vi "EXCOM-25-EQ.vi"(0 "VISA resource name":refnum<visa-resource-name>, 2 "Bool Refnum":refnum<vi>, 3 "Display Equinox":dbl format="%.2f") -> (5 "OK Done":bool, 6 "HA":dbl format="%<%H:%M:%S%0u>t", 7 "Q String":string, 8 "RA":dbl format="%<%H:%M:%S%0u>t", 9 "Rotateur":dbl format="%.2f", 10 "DEC":dbl format="%<%H:%M:%S%0u>t", 11 "Dome":dbl format="%.2f", 12 "Epoque":dbl format="%.2f", 13 "Focus":dbl format="%.2f", 14 "VISA resource name dup":refnum<visa-resource-name>, 15 "Masse d'air":dbl format="%.2f", 16 "Temps Sidéral":dbl format="%<%H:%M:%S%0u>t", 17 "Temps Universel":dbl format="%<%H:%M:%S%0u>t", 18 "Année":dbl format="%.2f", 19 "Error OUT":errorcluster)   [LabVIEW 2011]
panel:
  out "Response":string
  in  "Error IN":errorcluster
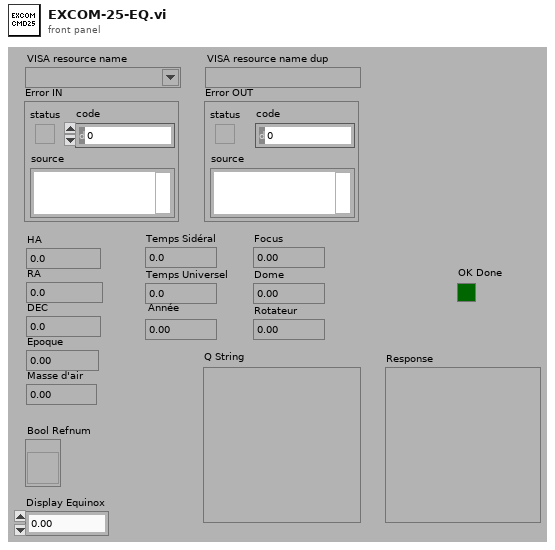
[diagram p1: front panel]
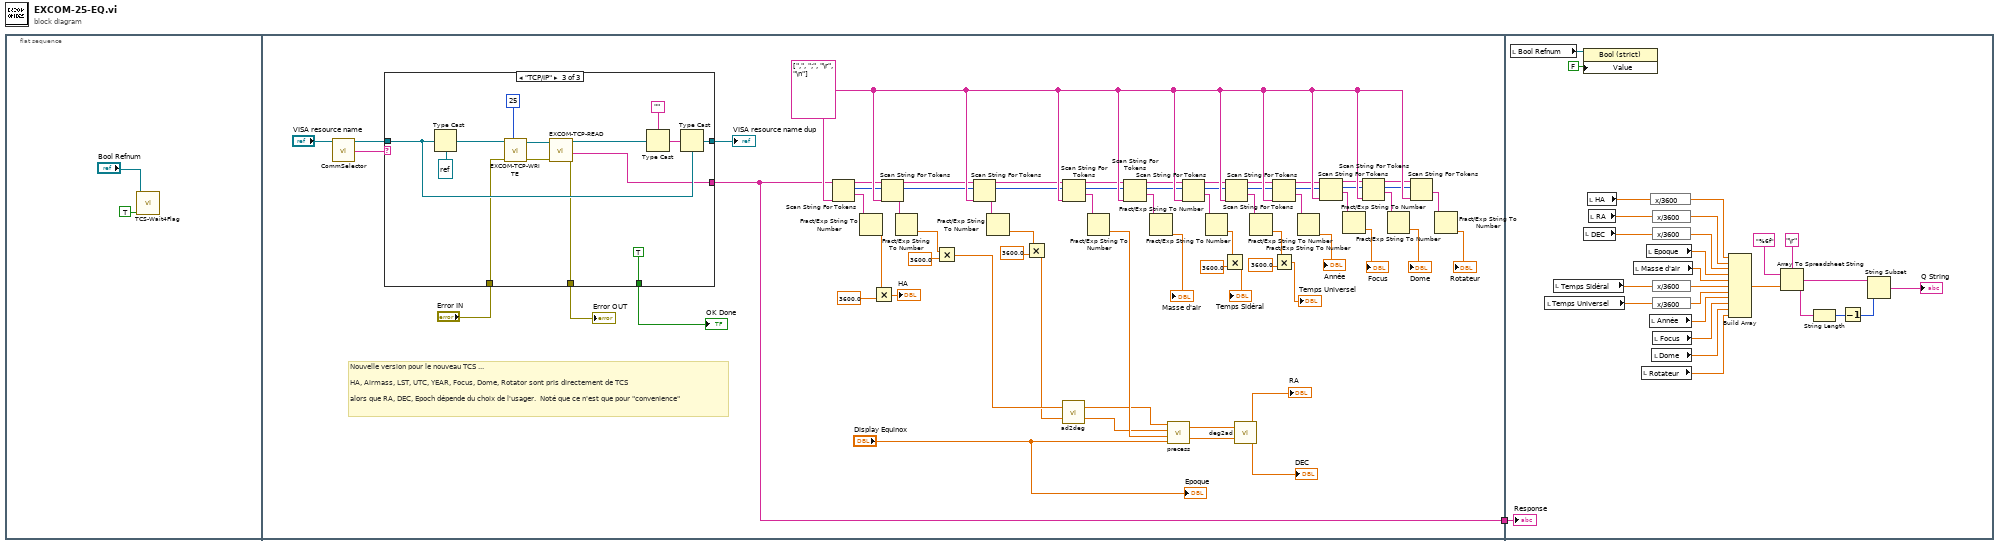
[diagram p0: block diagram]
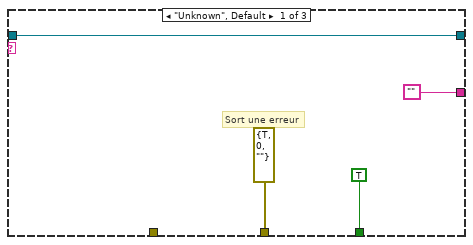
[diagram p2: hidden frame]
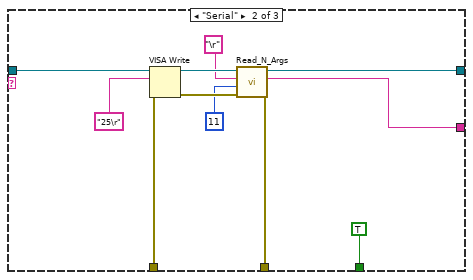
[diagram p3: hidden frame]
diagram:
  n1 = flat-sequence {
    tunnel: [w4] -> w1
    tunnel: w1 -> [w110]
    frame #0 {
      n2 = call "TCS-Wait4Flag.vi"("Raise Flag ?"=TRUE, "Ctl Refnum IN"="Bool Refnum") -> ()  [unwired: 8 in, 2 out]
    }
    frame #1 {
      w64 = string[] [",", ";", "\r", "\n"] ("delimiters (\\s,\\t,\\r,\\n)")
      # "Nouvelle version pour le nouveau TCS ...\n\nHA, Airmass, LST, UTC, YEAR, Focus, Dome, Rotator sont pris directement de TCS\n\nalors que RA, DEC, Epoch dépende du choix de l'usager.  Noté que ce n'est que pour \"convenience\""
      n3 = call "CommSelector.vi"("VISA resource name"="VISA resource name") -> ("VISA resource name"=w66:refnum<visa-resource-name>, "CommType"=w65:string)  [unwired: 13 in]
      n4 = case shown="\"TCP/IP\"" w65 {
        tunnel: w66 -> [w73 w78 w95]
        tunnel: [TRUE ("OK Done") TRUE ("OK Done") TRUE ("OK Done")] -> w71
        tunnel: [errorcluster {"status"=TRUE, "code"=0, "source"=""} ("error out") w85 w89] -> w70
        tunnel: [w73 w79 w94] -> w69
        tunnel: "Error IN" -> [_ w77 w90]
        tunnel: ["" w76 w87] -> w4
        frame "Unknown", Default {
          # "Sort une erreur"
        }
        frame "Serial" {
          n5 = VISA Write(VISA resource name=w78, write buffer="25\r" ("String to Send"), error in (no error)=w77) -> (VISA resource name out=w83:refnum<visa-resource-name>, error out=w84:errorcluster)  [unwired: 1 out]
          n6 = call "Read_N_Args.vi"("Error IN"=w84, "Nb_Args"=11, "Arg_Char"="\r", "VRN IN"=w83) -> ("Error OUT"=w85:errorcluster, "Answer"=w76:string, "VRN OUT"=w79:refnum<visa-resource-name>)  [unwired: 4 in, 1 out]
        }
        frame "TCP/IP" {
          n7 = Type Cast(type=refnum<k5> refnum ("CID Out"), x=w95) -> (*(type *) &x=w96:refnum<k5>)
          n8 = call "EXCOM-TCP-WRITE.vi"("Commande #"=25, "Error IN"=w90, "connection ID"=w96) -> ("Error OUT"=w100:errorcluster, "connection ID out"=w99:refnum<k5>)  [unwired: 4 in, 2 out]
          n9 = call "EXCOM-TCP-READ.vi"("Error In"=w100, "connection ID"=w99) -> ("Error Out"=w89:errorcluster, "Response"=w87:string, "CID Out"=w93:refnum<k5>)  [unwired: 5 in]
          n10 = Type Cast(type="", x=w93) -> (*(type *) &x=w91:string)
          n11 = Type Cast(type=w95, x=w91) -> (*(type *) &x=w94:refnum<visa-resource-name>)
        }
      }
      "VISA resource name dup" <- w69
      "OK Done" <- w71
      "Error OUT" <- w70
      n12 = Scan String For Tokens(6:w64, 9:w4) -> (1:w23:string, 2:w22:i32, 3:w21:string)  [unwired: 4 in, 1 out]
      n13 = Fract/Exp String To Number(string=w23) -> (number=w24:dbl)  [unwired: 3 in, 1 out]
      n14 = Multiply(x=w24, y=3600.0) -> (x*y=→"HA":dbl)
      n15 = Scan String For Tokens(6:w64, 8:w22, 9:w21) -> (1:w63:string, 2:w19:i32, 3:w20:string)  [unwired: 3 in, 1 out]
      n16 = Fract/Exp String To Number(string=w63) -> (number=w31:dbl)  [unwired: 3 in, 1 out]
      n17 = Multiply(x=w31, y=3600.0) -> (x*y=w13:dbl)
      n18 = Scan String For Tokens(6:w64, 8:w19, 9:w20) -> (1:w28:string, 2:w17:i32, 3:w18:string)  [unwired: 3 in, 1 out]
      n19 = Fract/Exp String To Number(string=w28) -> (number=w33:dbl)  [unwired: 3 in, 1 out]
      n20 = Multiply(x=w33, y=3600.0) -> (x*y=w12:dbl)
      n21 = call "ad2deg.vi"("DEC (sec)"=w12, "RA (sec)"=w13) -> ("DEC (°)"=w10:dbl, "RA (°)"=w11:dbl)
      n22 = Scan String For Tokens(6:w64, 8:w17, 9:w18) -> (1:w29:string, 2:w15:i32, 3:w16:string)  [unwired: 3 in, 1 out]
      n23 = Fract/Exp String To Number(string=w29) -> (number=w14:dbl)  [unwired: 3 in, 1 out]
      n24 = Scan String For Tokens(6:w64, 8:w15, 9:w16) -> (1:w30:string, 2:w61:i32, 3:w43:string)  [unwired: 3 in, 1 out]
      n25 = Fract/Exp String To Number(string=w30) -> (number=→"Masse d'air":dbl)  [unwired: 3 in, 1 out]
      n26 = call "precess.vi"("Eq2"="Display Equinox", "Eq1"=w14, "DEC 1"=w10, "RA 1"=w11) -> ("DEC 2"=w8:dbl, "RA 2"=w9:dbl)
      n27 = Scan String For Tokens(6:w64, 8:w61, 9:w43) -> (1:w38:string, 2:w40:i32, 3:w39:string)  [unwired: 3 in, 1 out]
      n28 = Fract/Exp String To Number(string=w38) -> (number=w35:dbl)  [unwired: 3 in, 1 out]
      n29 = Multiply(x=w35, y=3600.0) -> (x*y=→"Temps Sidéral":dbl)
      n30 = Scan String For Tokens(6:w64, 8:w40, 9:w39) -> (1:w37:string, 2:w42:i32, 3:w41:string)  [unwired: 3 in, 1 out]
      n31 = call "deg2ad.vi"("DEC (°)"=w8, "RA (°)"=w9) -> ("DEC (°)"=→"DEC":dbl, "RA (sec)"=→"RA":dbl)
      n32 = Fract/Exp String To Number(string=w37) -> (number=w34:dbl)  [unwired: 3 in, 1 out]
      n33 = Scan String For Tokens(6:w64, 8:w42, 9:w41) -> (1:w36:string, 2:w62:i32, 3:w53:string)  [unwired: 3 in, 1 out]
      n34 = Multiply(x=w34, y=3600.0) -> (x*y=→"Temps Universel":dbl)
      n35 = Fract/Exp String To Number(string=w36) -> (number=→"Année":dbl)  [unwired: 3 in, 1 out]
      n36 = Scan String For Tokens(6:w64, 8:w62, 9:w53) -> (1:w50:string, 2:w48:i32, 3:w49:string)  [unwired: 3 in, 1 out]
      n37 = Fract/Exp String To Number(string=w50) -> (number=→"Focus":dbl)  [unwired: 3 in, 1 out]
      n38 = Scan String For Tokens(6:w64, 8:w48, 9:w49) -> (1:w51:string, 2:w46:i32, 3:w47:string)  [unwired: 3 in, 1 out]
      n39 = Fract/Exp String To Number(string=w51) -> (number=→"Dome":dbl)  [unwired: 3 in, 1 out]
      n40 = Scan String For Tokens(6:w64, 8:w46, 9:w47) -> (1:w52:string)  [unwired: 3 in, 3 out]
      n41 = Fract/Exp String To Number(string=w52) -> (number=→"Rotateur":dbl)  [unwired: 3 in, 1 out]
      "Epoque" <- "Display Equinox"
    }
    frame #2 {
      n42 = local read "Bool Refnum"() -> (w126:refnum<vi>)
      n43 = local read "Temps Universel"() -> (w118:dbl)
      n44 = local read "Temps Sidéral"() -> (w119:dbl)
      n45 = property on="Property Node" class="Bool (strict)"(reference=w126, "Value"=FALSE) -> ()  [unwired: 1 in, 2 out]
      n46 = local read "DEC"() -> (w122:dbl)
      n47 = local read "HA"() -> (w124:dbl)
      n48 = local read "RA"() -> (w123:dbl)
      n49 = local read "Masse d'air"() -> (w120:dbl)
      n50 = local read "Rotateur"() -> (w114:dbl)
      n51 = local read "Epoque"() -> (w121:dbl)
      n52 = local read "Année"() -> (w117:dbl)
      n53 = expression code="x/3600"(w124) -> (w107:dbl)
      n54 = local read "Dome"() -> (w115:dbl)
      n55 = expression code="x/3600"(w123) -> (w109:dbl)
      n56 = expression code="x/3600"(w122) -> (w108:dbl)
      n57 = expression code="x/3600"(w119) -> (w106:dbl)
      n58 = expression code="x/3600"(w118) -> (w105:dbl)
      n59 = local read "Focus"() -> (w116:dbl)
      n60 = Build Array(w107, w109, w108, w121, w120, w106, w105, w117, w116, w115, w114) -> (w113:dbl[])
      n61 = Array To Spreadsheet String(delimiter (Tab)="\r", array=w113, 3:"%6f" ("format string")) -> (spreadsheet string=w104:string)
      n62 = String Length(string=w104) -> (length=w103:i32)
      n63 = Decrement(x=w103) -> (x-1=w102:i32)
      n64 = String Subset(string=w104, length (rest)=w102) -> (substring=→"Q String":string)  [unwired: 1 in]
      "Response" <- w110
    }
  }
